vi "WPI_CameraAttributeIsAuto.vi"(7 "Attr Format":string="CameraAttributes::%s::Mode", 10 "Attr String":string, 11 "Camera Address In":string) -> (2 "Auto?":bool, 3 "Camera Address Out":string)   [LabVIEW 2017]
doc: "Identify whether a camera attribute mode is auto or not.\n\nThis software is licensed. Open the labview\\readme\\WPI Robotics Library Open Source License.txt file for more information."
uses:
  <vilib>/userdefined/High Color/IMAQdx.ctl
  <resource>/objmgr/imaqdx.rc
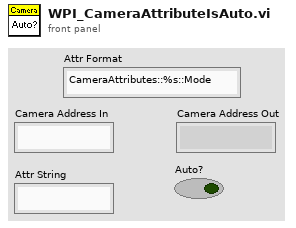
[diagram p1: front panel]
types:
  T1 = typedef "IMAQdx.ctl" = refnum<k21>
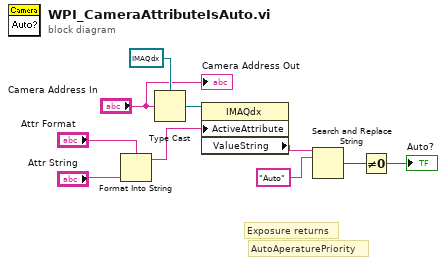
[diagram p0: block diagram]
diagram:
  # "Exposure returns"
  # "AutoAperaturePriority"
  n1 = Format Into String(format string="Attr Format", "Attr String") -> (resulting string=w7:string)  [unwired: 2 in, 1 out]
  n2 = Type Cast(type=T1 refnum ("Session In"), x="Camera Address In") -> (*(type *) &x=w10:T1)
  n3 = property class="IMAQdx"(reference=w10, "ActiveAttribute"=w7) -> ("ValueString"=w4:string)  [unwired: 1 in, 2 out]
  n4 = Search and Replace String(input string=w4, search string="Auto") -> (number of replacements=w2:i32)  [unwired: 6 in, 3 out]
  n5 = Not Equal To 0?(x=w2) -> (x != 0?=→"Auto?":bool)
  "Camera Address Out" <- "Camera Address In"
